vi "UTEX_Control_Enumerator.vi"(7 "Pulse Width (ns)":refnum<vi>, 8 "High Pass (MHz) Ref":refnum<vi>, 9 "Low Pass (MHz) Ref":refnum<vi>, 10 "Voltage (V) Ref":refnum<vi>, 11 "Gain (dB)":refnum<vi>) -> (0 "High Pass (MHz)":T2, 1 "Low Pass (MHz)":T2, 2 "Voltage (V)":T2, 3 "Gain (dB)":T3, 5 "Pulse Width (ns)":T1)   [LabVIEW 2022 SP3]
uses:
  <vilib>/Utility/miscctls.llb/LVStringsAndValuesArrayTypeDef_I32.ctl
  <vilib>/Utility/miscctls.llb/LVStringsAndValuesArrayTypeDef_U16.ctl
  <vilib>/Utility/miscctls.llb/LVStringsAndValuesArrayTypeDef_DBL.ctl
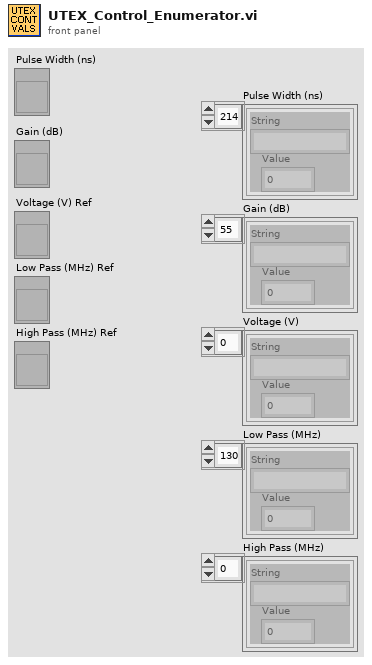
[diagram p1: front panel]
types:
  T1 = typedef "LVStringsAndValuesArrayTypeDef_DBL.ctl" = cluster{"String":string, "Value":dbl}[]
  T2 = typedef "LVStringsAndValuesArrayTypeDef_U16.ctl" = cluster{"String":string, "Value":u16}[]
  T3 = typedef "LVStringsAndValuesArrayTypeDef_I32.ctl" = cluster{"String":string, "Value":i32}[]
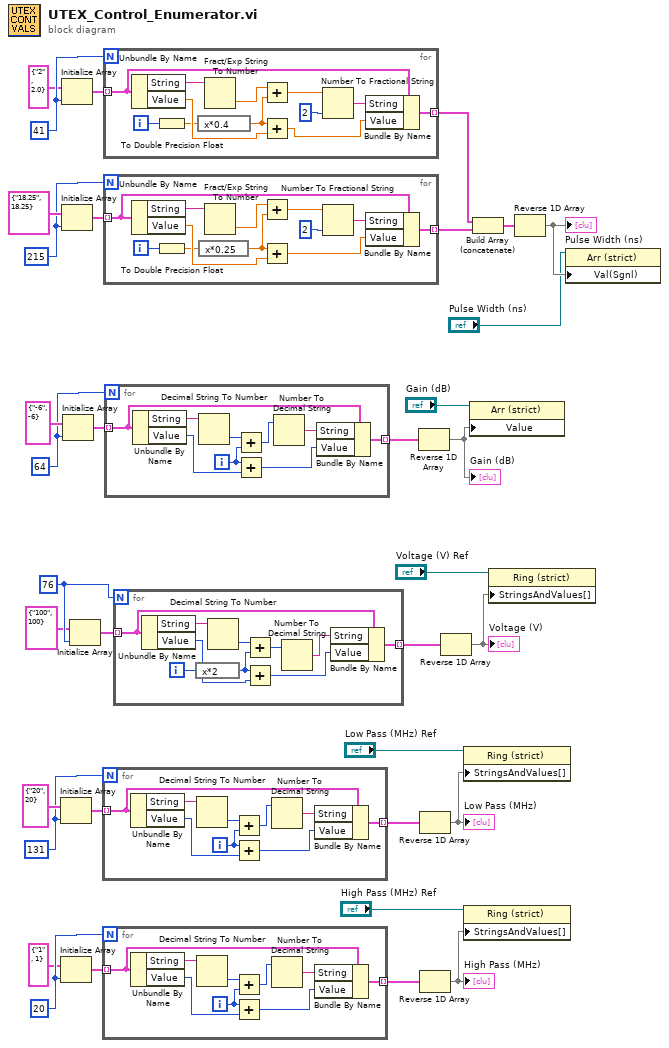
[diagram p0: block diagram]
diagram:
  w8 = 215
  w12 = 41
  w17 = 20
  w22 = 131
  w30 = 76
  w33 = 64
  n1 = Initialize Array(cluster{"String":string, "Value":i32} {"String"="20", "Value"=20}, w22) -> (w21:cluster{"String":string, "Value":i32}[])
  n2 = Initialize Array(cluster{"String":string, "Value":i32} {"String"="1", "Value"=1}, w17) -> (w18:cluster{"String":string, "Value":i32}[])
  n3 = Initialize Array(cluster{"String":string, "Value":dbl} {"String"="2", "Value"=2.0}, w12) -> (w13:cluster{"String":string, "Value":dbl}[])
  n4 = Initialize Array(cluster{"String":string, "Value":dbl} {"String"="18.25", "Value"=18.25}, w8) -> (w7:cluster{"String":string, "Value":dbl}[])
  n5 = Initialize Array(cluster{"String":string, "Value":i32} {"String"="-6", "Value"=-6}, w33) -> (w32:cluster{"String":string, "Value":i32}[])
  n6 = Initialize Array(cluster{"String":string, "Value":i32} {"String"="100", "Value"=100}, w30) -> (w31:cluster{"String":string, "Value":i32}[])
  n7 = for {
    N: w22 -> [_]
    tunnel: w21 -> [w44] mode=indexing
    tunnel: [w37] -> w24 mode=indexing
    i -> [w36]
    n8 = Unbundle By Name(w44) -> ("String"=w41:string, "Value"=w43:i32)
    n9 = Decimal String To Number(string=w41) -> (number=w39:i32)  [unwired: 2 in, 1 out]
    n10 = Add(x=w39, y=w36) -> (x+y=w38:i32)
    n11 = Add(x=w36, y=w43) -> (x+y=w42:i32)
    n12 = Number To Decimal String(number=w38) -> (decimal integer string=w40:string)  [unwired: 1 in]
    n13 = Bundle By Name(cluster=w44, "String"=w40, "Value"=w42) -> (w37:cluster{"String":string, "Value":i32})
  }
  n14 = for {
    N: w17 -> [_]
    tunnel: w18 -> [w53] mode=indexing
    tunnel: [w46] -> w15 mode=indexing
    i -> [w45]
    n15 = Unbundle By Name(w53) -> ("String"=w50:string, "Value"=w52:i32)
    n16 = Decimal String To Number(string=w50) -> (number=w48:i32)  [unwired: 2 in, 1 out]
    n17 = Add(x=w48, y=w45) -> (x+y=w47:i32)
    n18 = Add(x=w45, y=w52) -> (x+y=w51:i32)
    n19 = Number To Decimal String(number=w47) -> (decimal integer string=w49:string)  [unwired: 1 in]
    n20 = Bundle By Name(cluster=w53, "String"=w49, "Value"=w51) -> (w46:cluster{"String":string, "Value":i32})
  }
  n21 = for {
    N: w12 -> [_]
    tunnel: w13 -> [w65] mode=indexing
    tunnel: [w57] -> w10 mode=indexing
    i -> [w58]
    n22 = Unbundle By Name(w65) -> ("String"=w62:string, "Value"=w64:dbl)
    n23 = To Double Precision Float(number=w58) -> (double precision float=w55:dbl)
    n24 = expression code="x*0.4"(w55) -> (w56:dbl)
    n25 = Fract/Exp String To Number(string=w62) -> (number=w60:dbl)  [unwired: 3 in, 1 out]
    n26 = Add(x=w60, y=w56) -> (x+y=w59:dbl)
    n27 = Add(x=w56, y=w64) -> (x+y=w63:dbl)
    n28 = Number To Fractional String(number=w59, precision (6)=i16 2) -> (F-format string=w61:string)  [unwired: 2 in]
    n29 = Bundle By Name(cluster=w65, "String"=w61, "Value"=w63) -> (w57:cluster{"String":string, "Value":dbl})
  }
  n30 = for {
    N: w8 -> [_]
    tunnel: w7 -> [w77] mode=indexing
    tunnel: [w69] -> w5 mode=indexing
    i -> [w70]
    n31 = Unbundle By Name(w77) -> ("String"=w74:string, "Value"=w76:dbl)
    n32 = To Double Precision Float(number=w70) -> (double precision float=w67:dbl)
    n33 = expression code="x*0.25"(w67) -> (w68:dbl)
    n34 = Fract/Exp String To Number(string=w74) -> (number=w72:dbl)  [unwired: 3 in, 1 out]
    n35 = Add(x=w72, y=w68) -> (x+y=w71:dbl)
    n36 = Add(x=w68, y=w76) -> (x+y=w75:dbl)
    n37 = Number To Fractional String(number=w71, precision (6)=i16 2 ("width (-)")) -> (F-format string=w73:string)  [unwired: 2 in]
    n38 = Bundle By Name(cluster=w77, "String"=w73, "Value"=w75) -> (w69:cluster{"String":string, "Value":dbl})
  }
  n39 = for {
    N: w33 -> [_]
    tunnel: w32 -> [w86] mode=indexing
    tunnel: [w78] -> w28 mode=indexing
    i -> [w79]
    n40 = Unbundle By Name(w86) -> ("String"=w83:string, "Value"=w85:i32)
    n41 = Decimal String To Number(string=w83) -> (number=w81:i32)  [unwired: 2 in, 1 out]
    n42 = Add(x=w81, y=w79) -> (x+y=w80:i32)
    n43 = Add(x=w79, y=w85) -> (x+y=w84:i32)
    n44 = Number To Decimal String(number=w80) -> (decimal integer string=w82:string)  [unwired: 1 in]
    n45 = Bundle By Name(cluster=w86, "String"=w82, "Value"=w84) -> (w78:cluster{"String":string, "Value":i32})
  }
  n46 = for {
    N: w30 -> [_]
    tunnel: w31 -> [w96] mode=indexing
    tunnel: [w88] -> w27 mode=indexing
    i -> [w89]
    n47 = Unbundle By Name(w96) -> ("String"=w93:string, "Value"=w95:i32)
    n48 = expression code="x*2"(w89) -> (w87:i32)
    n49 = Decimal String To Number(string=w93) -> (number=w91:i32)  [unwired: 2 in, 1 out]
    n50 = Add(x=w91, y=w87) -> (x+y=w90:i32)
    n51 = Add(x=w87, y=w95) -> (x+y=w94:i32)
    n52 = Number To Decimal String(number=w90) -> (decimal integer string=w92:string)  [unwired: 1 in]
    n53 = Bundle By Name(cluster=w96, "String"=w92, "Value"=w94) -> (w88:cluster{"String":string, "Value":i32})
  }
  n54 = Reverse 1D Array(array=w28) -> (reversed array=w3:cluster{"String":string, "Value":i32}[])
  "Gain (dB)" <- w3
  n55 = Reverse 1D Array(array=w24) -> (reversed array=w25:cluster{"String":string, "Value":i32}[])
  "Low Pass (MHz)" <- w25
  n56 = Reverse 1D Array(array=w15) -> (reversed array=w14:cluster{"String":string, "Value":i32}[])
  "High Pass (MHz)" <- w14
  n57 = Reverse 1D Array(array=w27) -> (reversed array=w26:cluster{"String":string, "Value":i32}[])
  "Voltage (V)" <- w26
  n58 = property class="Ring (strict)"(reference="Low Pass (MHz) Ref", "StringsAndValues[]"=w25) -> ()  [unwired: 1 in, 2 out]
  n59 = property class="Ring (strict)"(reference="High Pass (MHz) Ref", "StringsAndValues[]"=w14) -> ()  [unwired: 1 in, 2 out]
  n60 = property class="Arr (strict)"(reference="Gain (dB)", "Value"=w3) -> ()  [unwired: 1 in, 2 out]
  n61 = Build Array (concatenate)(w10, w5) -> (w6:cluster{"String":string, "Value":dbl}[])
  n62 = property class="Ring (strict)"(reference="Voltage (V) Ref", "StringsAndValues[]"=w26) -> ()  [unwired: 1 in, 2 out]
  n63 = Reverse 1D Array(array=w6) -> (reversed array=w2:cluster{"String":string, "Value":dbl}[])
  "Pulse Width (ns)" <- w2
  n64 = property class="Arr (strict)"(reference="Pulse Width (ns)", "Val(Sgnl)"=w2) -> ()  [unwired: 1 in, 2 out]
